vi "Release Lock.vi"(8 "error in (no error)":errorcluster, 9 "timeout (0 ms)":i32 format="%d ms", 10 "new lock status (T)":bool=TRUE, 11 "Protected Pointer in":refnum<class "Protected Pointer.lvclass">) -> (0 "error out":errorcluster, 1 "timed out?":bool, 3 "Protected Pointer out":refnum<class "Protected Pointer.lvclass">)   [LabVIEW 2016, in "Memory Manager.lvlib" / "Protected Pointer.lvclass"]
uses:
  Lockable Pointer/Protected Pointer.lvclass
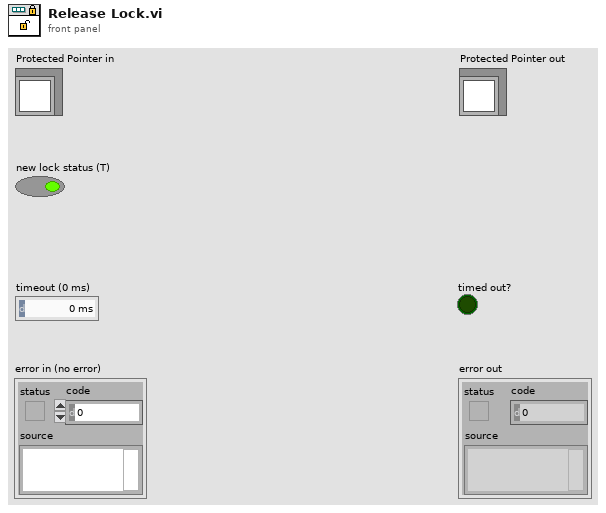
[diagram p1: front panel]
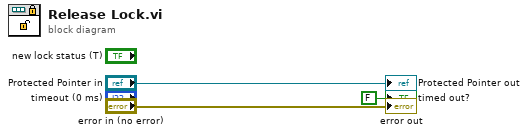
[diagram p0: block diagram]
diagram:
  "error out" <- "error in (no error)"
  "Protected Pointer out" <- "Protected Pointer in"
  "timed out?" <- FALSE ("timed out?")
